vi "Romi-Drive-System-Globals.vi"() -> ()   [LabVIEW 2019]
panel:
  out "Drive_Gyro_Raw":dbl
  out "Drive_Right_Motor":dbl
  out "Drive_Left_Motor":dbl
  out "Drive_Right_Dist":dbl
  out "Drive_Left_Dist":dbl
  out "Drive_Right_Speed_Filt":dbl
  out "Drive_Left_Speed_Filt":dbl
  out "Drive_Right_Speed":dbl
  out "Drive_Left_Speed":dbl
  out "Drive_Right_Dmd":dbl
  out "Drive_Left_Dmd":dbl
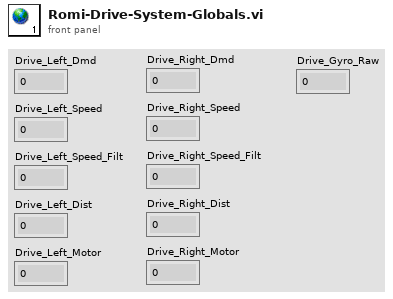
[diagram p1: front panel]
diagram:
